vi "ex3-2.vi"() -> ()   [LabVIEW 2009]
panel:
  out "文字輸出":string
  in  "文字輸入":string
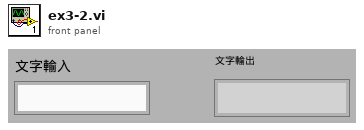
[diagram p1: front panel]
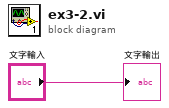
[diagram p0: block diagram]
diagram:
  "文字輸出" <- "文字輸入"
